vi "State_Machine.vi"(8 "error in (no error)":errorcluster caption="entrée d'erreur (pas d'erreur)", 11 "Delay en entrée":refnum<class "Enter_Qr_P2056.lvclass">) -> (0 "error out":errorcluster caption="sortie d'erreur", 2 "Json_String":string, 3 "Delay en sortie":refnum<class "Enter_Qr_P2056.lvclass">)   [LabVIEW 2020, in "Library Test.lvlib" / "Enter_Qr_P2056.lvclass"]
uses:
  Enter_Qr_P2056.lvclass
  C:/Users/ngarcin/OneDrive - Altyor/Standard TB/Class/Test/Test (Default)/Test (Default).lvclass
  Popup/Class Popup Operator_Input QR_P2056/Class Popup Operator_Input QR_P2056.lvclass
  C:/Users/ngarcin/OneDrive - Altyor/Standard TB/Class/Popup/Class Popup (Main)/Class Popup (Main).lvclass
  Enter_Qr_P2056.lvclass/Enter_Qr_P2056.ctl
  JSON API/Variant JSON/Variant JSON.lvlib
  JSON API/Get Polymorphic/JSON GetSet.lvlib
  JSON API/JSON Value/Set from JSON string.vi
  JSON API/JSON Value/JSON Value.lvclass
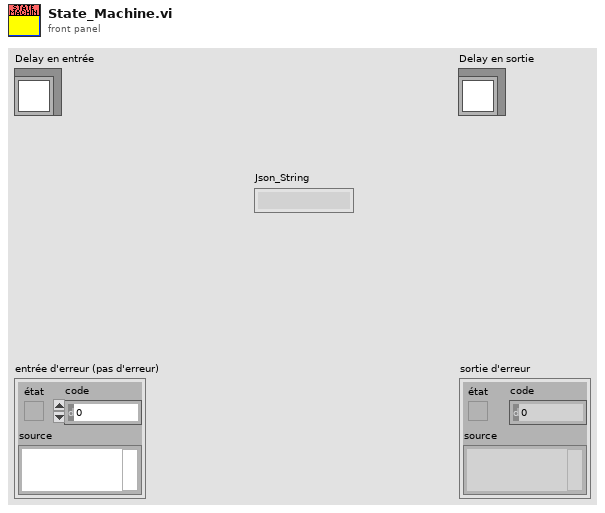
[diagram p1: front panel]
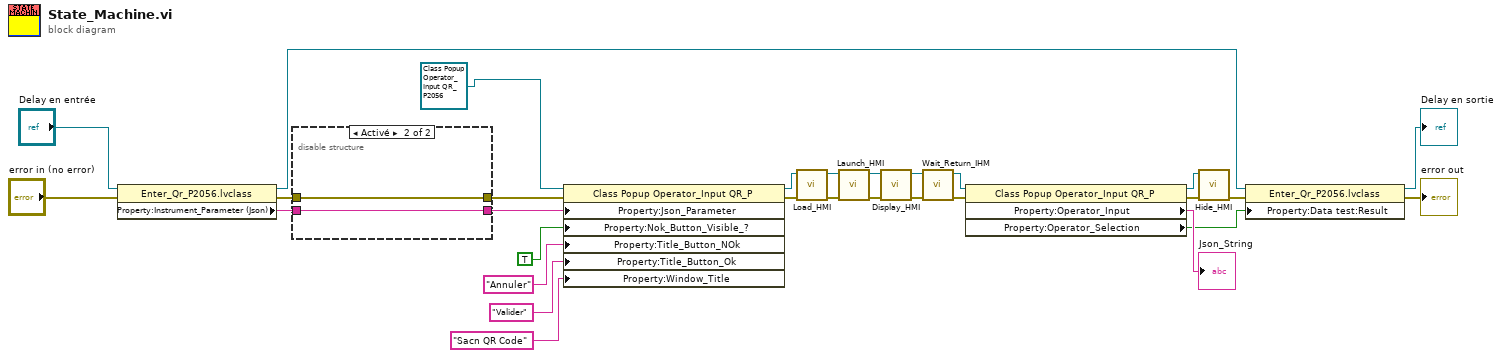
[diagram p0: block diagram]
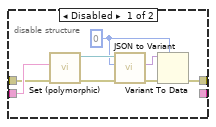
[diagram p2: hidden frame]
diagram:
  n1 = property class="Enter_Qr_P2056.lvclass"(reference="Delay en entrée", error in="error in (no error)") -> (reference out=w6:refnum<class "Enter_Qr_P2056.lvclass">, error out=w26:errorcluster, "Property:Instrument_Parameter (Json)"=w28:string)
  n2 = disable-structure shown="Activé" {
    disable-tunnel: w28 -> [w32 w38]
    disable-tunnel: w26 -> [w31 w39]
    disable-tunnel: [w30 w39] -> w13
    disable-tunnel: [_ w38] -> w9
    frame Disabled {
      w33 = u32 0 ("Channel")
      n3 = call-poly "Set (polymorphic).vi"("error in (no error)"=w31, "JSON stream"=w32) -> ("error out"=w35:errorcluster, "JSON Value out"=w37:refnum<class "JSON Value.lvclass">)  [unwired: 7 in, 1 out]
      n4 = call "JSON to Variant.vi"("error in (no error)"=w35, "Variant (Data Type)"=w33, "JSON Value"=w37) -> ("error out"=w36:errorcluster, "Variant out"=w34:variant)  [unwired: 7 in]
      n5 = Variant To Data(error in=w36, type=w33, Variant=w34) -> (error out=w30:errorcluster)  [unwired: 1 out]
    }
    frame Enabled {
    }
  }
  n6 = property class="Class Popup Operator_Input QR_P"(reference=refnum<class "Class Popup Operator_Input QR_P2056.lvclass"> refnum ("Library Popup.lvlib:Class Popup Operator_Input QR_P2056.lvclass"), error in=w13, "Property:Json_Parameter"=w9, "Property:Nok_Button_Visible_?"=TRUE ("Nok_Button_Visible_?"), "Property:Title_Button_NOk"="Annuler" ("Title_Button_NOk"), "Property:Title_Button_Ok"="Valider" ("Title_Button_Ok"), "Property:Window_Title"="Sacn QR Code" ("Window_Title")) -> (reference out=w19:refnum<class "Class Popup Operator_Input QR_P2056.lvclass">, error out=w18:errorcluster)
  n7 = call-dynamic "Load_HMI.vi"("error in (no error)"=w18, "Class Popup (Default) en entrée"=w19) -> ("error out"=w25:errorcluster, "Class Popup (Default) en sortie"=w24:refnum<class "Class Popup Operator_Input QR_P2056.lvclass">)  [unwired: 8 in]
  n8 = call-dynamic "Launch_HMI.vi"("error in (no error)"=w25, "Class Popup (Default) en entrée"=w24) -> ("error out"=w23:errorcluster, "Class Popup (Default) en sortie"=w21:refnum<class "Class Popup Operator_Input QR_P2056.lvclass">)  [unwired: 8 in]
  n9 = call-dynamic "Display_HMI.vi"("error in (no error)"=w23, "Class Popup (Default) en entrée"=w21) -> ("error out"=w22:errorcluster, "Class Popup (Default) en sortie"=w20:refnum<class "Class Popup Operator_Input QR_P2056.lvclass">)  [unwired: 8 in]
  n10 = call-dynamic "Wait_Return_IHM.vi"("error in (no error)"=w22, "Class Popup (Default) en entrée"=w20) -> ("error out"=w14:errorcluster, "Class Popup (Default) en sortie"=w15:refnum<class "Class Popup Operator_Input QR_P2056.lvclass">)  [unwired: 8 in]
  n11 = property class="Class Popup Operator_Input QR_P"(reference=w15, error in=w14) -> (reference out=w8:refnum<class "Class Popup Operator_Input QR_P2056.lvclass">, error out=w7:errorcluster, "Property:Operator_Input"=→"Json_String":string, "Property:Operator_Selection"=w4:bool)
  n12 = call-dynamic "Hide_HMI.vi"("error in (no error)"=w7, "Class Popup (Default) en entrée"=w8) -> ("error out"=w5:errorcluster)  [unwired: 8 in, 1 out]
  n13 = property class="Enter_Qr_P2056.lvclass"(reference=w6, error in=w5, "Property:Data test:Result"=w4) -> (reference out=→"Delay en sortie":refnum<class "Enter_Qr_P2056.lvclass">, error out=→"error out":errorcluster)
